vi "数据库操作.vi"(6 "返回数据":bool, 8 "error in (no error)":errorcluster, 10 "SQL query":string) -> (0 "error out":errorcluster, 2 "recordset data":variant[][](array[variant]))   [LabVIEW 2015]
uses:
  <vilib>/addons/database/Connection.llb/DB Tools Open Connec (String).vi
  <vilib>/addons/database/Connection.llb/Conn Execute.vi
  <vilib>/addons/database/Recordset.llb/Rec Fetch Recordset Data (R).vi
  <vilib>/addons/database/Recordset.llb/Rec Destroy - Connection.vi
  <vilib>/addons/database/NI_Database_API.lvlib
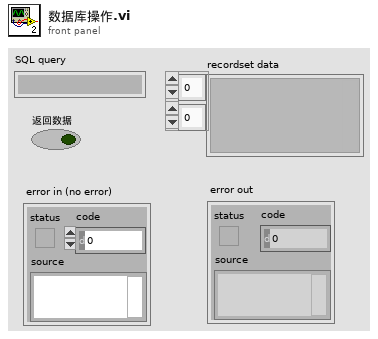
[diagram p1: front panel]
types:
  T1 = typedef "NI_Database_API.lvlib/Conn ObjectReference.ctl" = refnum<k1>
  T2 = typedef "NI_Database_API.lvlib/Rec ObjectReference.ctl" = refnum<k1>
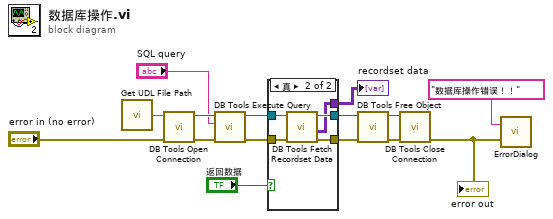
[diagram p0: block diagram]
diagram:
  n1 = call "Get UDL File Path.vi"() -> ("connection information"=w13:string)
  n2 = call-poly <vilib>:"DB Tools Open Connection.vi"("error in (no error)"="error in (no error)", "connection information"=w13) -> ("error out"=w14:errorcluster, "connection reference"=w15:T1)  [unwired: 6 in]
  n3 = call-poly <vilib>:"DB Tools Execute Query.vi"("error in (no error)"=w14, "SQL query"="SQL query", "connection reference"=w15) -> ("error out"=w10:errorcluster, "recordset reference"=w11:T2)  [unwired: 5 in]
  n4 = case shown="真" "返回数据" {
    tunnel: w11 -> [w16 w22]
    tunnel: w10 -> [w17 w21]
    tunnel: [w17 w20] -> w9
    tunnel: [w16 w19] -> w8
    tunnel: [_ w18] -> w5
    frame False {
    }
    frame True {
      n5 = call-poly <vilib>:"DB Tools Fetch Recordset Data.vi"("error in (no error)"=w21, "recordset reference"=w22) -> ("error out"=w20:errorcluster, "recordset data"=w18:variant[][], "recordset reference out"=w19:T2)  [unwired: 3 in]
    }
  }
  "recordset data" <- w5
  n6 = call-poly <vilib>:"DB Tools Free Object.vi"("error in (no error)"=w9, "recordset reference"=w8) -> ("error out"=w6:errorcluster, "connection reference"=w12:T1)  [unwired: 8 in]
  n7 = call <vilib>:"DB Tools Close Connection.vi"("error in (no error)"=w6, "connection reference"=w12) -> ("error out"=w2:errorcluster)  [unwired: 5 in]
  "error out" <- w2
  n8 = call "ErrorDialog.vi"("error in"=w2, "message"="数据库操作错误！！") -> ()  [unwired: 1 in]
